vi "Plane Coordinate Generator.vi"(8 "error in (no error)":errorcluster, 10 "AcquireZplane Index":i32, 11 "AOL_Globals":T1={"Imaging Protocol"=enum."AOL Z-Stack", "Number of POI"=0, "Number of Miniscans"=0, "Number of Trials"=0, "Number of Cycles "=0, "# Averaged Frames"=0, "Laser power (%)"=0, "Pockels (V)"=0.0, "Acquisition Length (sec)"=0.0, "Fill time (us)"=0.0, "POI Dwell time (us)"=0.0, "Miniscan Dwell time per pixel (us)"=0.0, "PMT 1"=0.0, "PMT 2"=0.0, "Back Apperture (mA)"=512.0, "Frame Size"=0, "Center Frequency"=0.0, "Field of View (um)"=175.0, "Field of View (norm)"=0.0, "DwellTime (us)"=0.0, "Ref Dwell Time (us)"=0.0, "Wavelength (nm)"=0.0, "Zoom"=0.0, "AOL Z"=0.0, "AOL Mode"=enum."Raster", "GridXY"=0.0, "GridZ"=0.0, "TriggerPeriod (sec)"=0.0, "Number of Pixels in Miniscan"=0, "Experiment folder path"=path "", "X centre"=0.0, "Y centre"=0.0, "Angle (degrees)"=0.0, "Angle Xs (degrees)"=0.0, "Angle Ys (degrees)"=0.0, "Plane Mode"=0, "Threshold"=[], "Regenerate Chirps"=FALSE, "Rectangle ROI length (pixels)"=0, "Rectangle ROI height (pixels)"=0, "AOD fill"=4900, "StartupDelay"=0, "Samples Wait after Trigger"=5080, "Slip Cycle"=600000, "Add Cycle"=TRUE, "Functional Mode"=enum."Point", "Z Start"=0.0, "Z Stop"=0.0, "# Planes"=0, "Total Pixels"=0, "Variable Miniscan Pixels"=[], "Use Variable Length"=FALSE, "Use Variable Resolution"=FALSE, "Laser power (%) at Z Start"=0, "Laser power (%) at Z Stop"=0, "Ref Z Step"=0} {"Angle Ys (degrees)" format="%#.6g"; "Angle Xs (degrees)" format="%#.6g"; "Plane Mode" items=["XY Plane", "XZ Plane", "YZ Plane", "arbitraryplane"]; "Frame Size" items=["100X100"=100, "128X128"=128, "200X200"=200, "256X256"=256, "512X512"=512, "1024x1024"=1024, "2048x2048"=2048]; "Back Apperture (mA)" format="%#.6g"; "Pockels (V)" format="%#.6g"; "PMT 2" format="%#.6g"; "PMT 1" format="%#.6g"; "Angle (degrees)" format="%#.6g"; "POI Dwell time (us)" format="%#.6g"}) -> (0 "error out":errorcluster, 3 "ROI Attributes (broken down to miniscans)":T7)   [LabVIEW 2020]
uses:
  Typedefs/ROI XY coordinates cluster.ctl
  Typedefs/Controls/AOL_Globals.ctl
  Typedefs/Imaging Protocols enum.ctl
  Typedefs/Frame Size.ctl
  Typedefs/AOL modes.ctl
  Typedefs/Plane Mode.ctl
  Typedefs/Functional Mode.ctl
  User Interface/Visualisation/Functional Imaging Viewer/Typedefs/ROI parameters data type.ctl
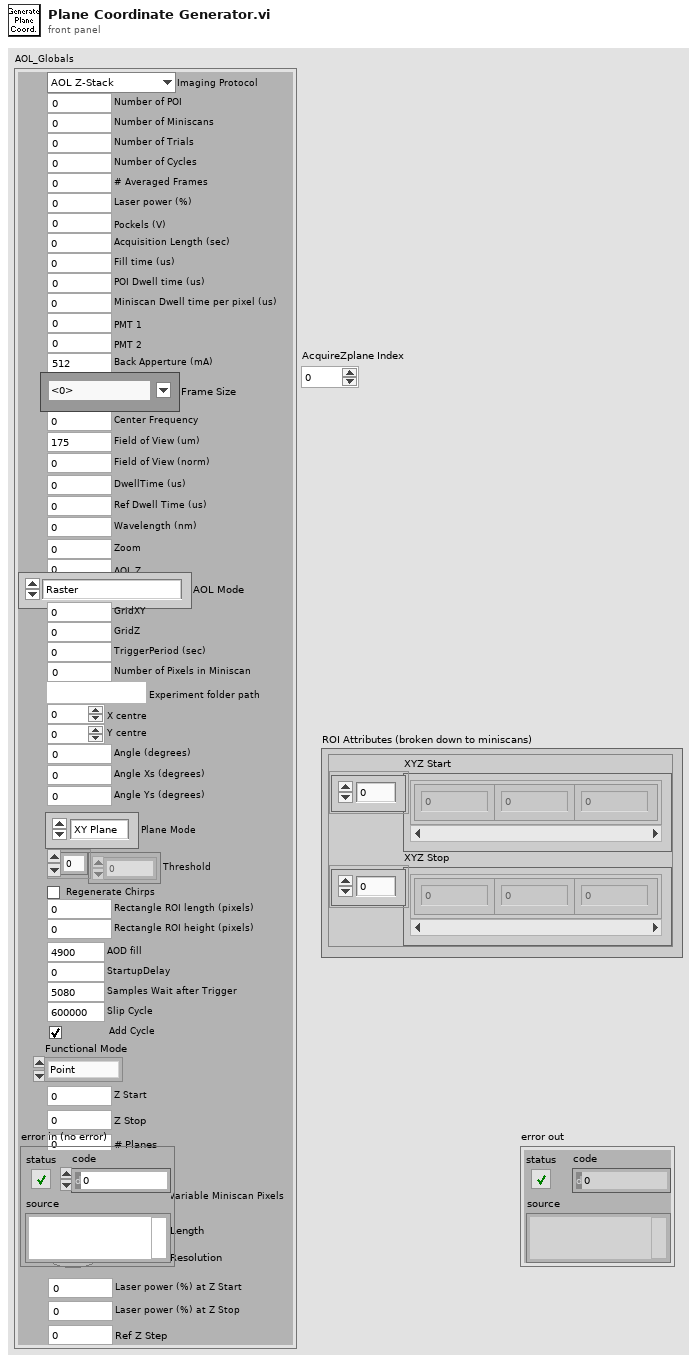
[diagram p1: front panel]
types:
  T1 = typedef "AOL_Globals.ctl" = cluster{"Imaging Protocol":T2, "Number of POI":u16, "Number of Miniscans":u16, "Number of Trials":u16, "Number of Cycles ":u64, "# Averaged Frames":u16, "Laser power (%)":u8, "Pockels (V)":dbl, "Acquisition Length (sec)":dbl, "Fill time (us)":dbl, "POI Dwell time (us)":dbl, "Miniscan Dwell time per pixel (us)":dbl, "PMT 1":dbl, "PMT 2":dbl, "Back Apperture (mA)":dbl, "Frame Size":T3, "Center Frequency":dbl, "Field of View (um)":dbl, "Field of View (norm)":dbl, "DwellTime (us)":dbl, "Ref Dwell Time (us)":dbl, "Wavelength (nm)":dbl, "Zoom":dbl, "AOL Z":dbl, "AOL Mode":T4, "GridXY":dbl, "GridZ":dbl, "TriggerPeriod (sec)":dbl, "Number of Pixels in Miniscan":u16, "Experiment folder path":path, "X centre":dbl, "Y centre":dbl, "Angle (degrees)":dbl, "Angle Xs (degrees)":dbl, "Angle Ys (degrees)":dbl, "Plane Mode":T5, "Threshold":u16[], "Regenerate Chirps":bool, "Rectangle ROI length (pixels)":u16, "Rectangle ROI height (pixels)":u16, "AOD fill":u16, "StartupDelay":i32, "Samples Wait after Trigger":u16, "Slip Cycle":u32, "Add Cycle":bool, "Functional Mode":T6, "Z Start":dbl, "Z Stop":dbl, "# Planes":i32, "Total Pixels":i32, "Variable Miniscan Pixels":u16[], "Use Variable Length":bool, "Use Variable Resolution":bool, "Laser power (%) at Z Start":u8, "Laser power (%) at Z Stop":u8, "Ref Z Step":i8}
  T2 = typedef "Imaging Protocols enum.ctl" = enum16{"AOL Z-Stack", "Motor Z Stack", "Parameter Sweep", "Functional Acquisition", "Single Plane Acquisition", "Volume Acquisition", "Live Imaging", "Live Plane Imaging", "Live Volume Imaging"}
  T3 = typedef "Frame Size.ctl" = u16
  T4 = typedef "AOL modes.ctl" = enum16{"Raster", "Structural", "Pointing", "Mini Scan", "Alignment"}
  T5 = typedef "Plane Mode.ctl" = u16
  T6 = typedef "Functional Mode.ctl" = enum16{"Point", "Line", "Patch", "Plane", "Volume"}
  T7 = typedef "ROI XY coordinates cluster.ctl" = cluster{"XYZ Start":cluster{"X":sgl, "Y":sgl, "Z":sgl}[], "XYZ Stop":cluster{"X":sgl, "Y":sgl, "Z":sgl}[]}
  T8 = typedef "ROI parameters data type.ctl" = cluster{"ROI index":dbl, "ROI ID":dbl, "ROI Time (ns)":dbl, "Pixels in ROI":dbl, "X start":dbl, "Y start":dbl, "Z start":dbl, "X stop":dbl, "Y stop":dbl, "Z stop":dbl, "Angle (deg)":dbl, "Composite ID":dbl, "Number of lines":dbl, "Frame Size":dbl, "Zoom":dbl, "Laser Power (%)":dbl, "ROI group ID":dbl, "Resolution":dbl, "Dwell Time per pixel":dbl, "Pixels per miniscan":dbl, "Original FOV (um)":dbl, "Apparent Frame Size":dbl, "Z Plane Idx":i32[], "Z Plane codes":i32[]}
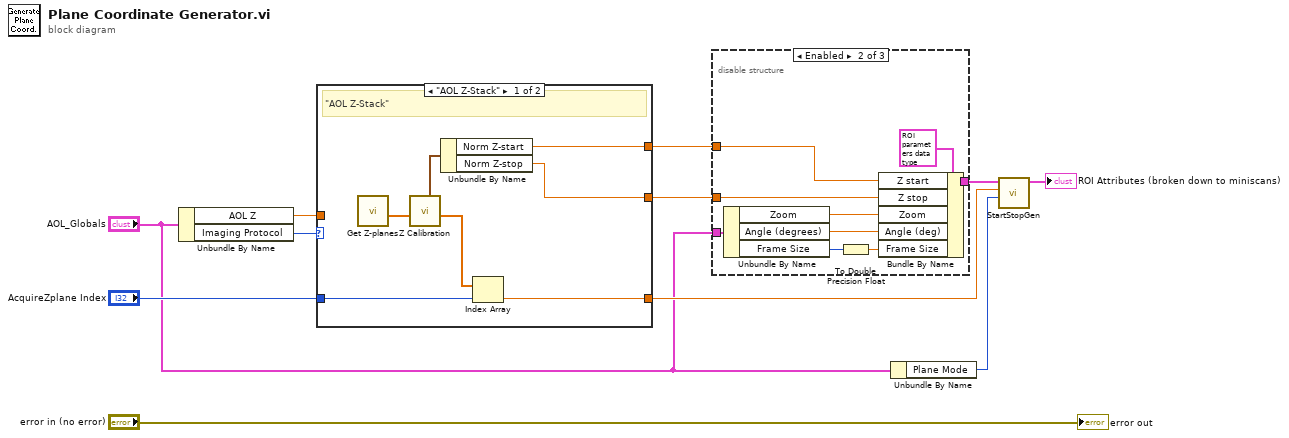
[diagram p0: block diagram]
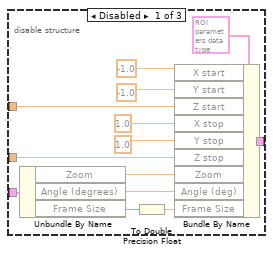
[diagram p2: hidden frame]
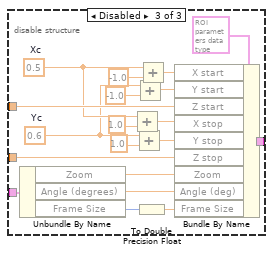
[diagram p3: hidden frame]
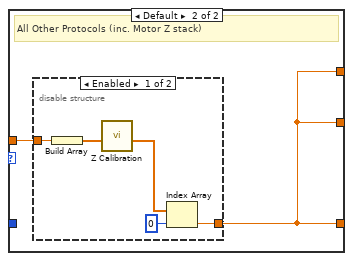
[diagram p4: hidden frame]
diagram:
  n1 = Unbundle By Name("AOL_Globals") -> ("AOL Z"=w3:dbl, "Imaging Protocol"=w4:T2)
  n2 = case shown="\"AOL Z-Stack\"" w4 {
    tunnel: [w12 w20] -> w10
    tunnel: [w13 w20] -> w9
    tunnel: "AcquireZplane Index" -> [w18 _]
    tunnel: [w17 w20] -> w6
    tunnel: w3 -> [_ w19]
    frame "AOL Z-Stack" {
      # "\"AOL Z-Stack\""
      n3 = call "Get Z-planes.vi"() -> ("Z Planes(um)"=w16:dbl[])  [unwired: 7 in, 4 out]
      n4 = call "Z Calibration.vi"("Z Planes"=w16) -> ("Norm Z"=w15:dbl[], "Norm Z start/stop"=w14:cluster{"Norm Z-start":dbl, "Norm Z-stop":dbl})  [unwired: 7 in, 2 out]
      n5 = Unbundle By Name(w14) -> ("Norm Z-start"=w13:dbl, "Norm Z-stop"=w12:dbl)
      n6 = Index Array(array=w15, index=w18) -> (element=w17:dbl)
    }
    frame Default {
      # "All Other Protocols (inc. Motor Z stack)"
      n7 = disable-structure shown="Enabled" {
        disable-tunnel: [w22 w26] -> w20
        disable-tunnel: w19 -> [w21 w26]
        frame Enabled {
          n8 = Build Array(w21) -> (w25:dbl[])
          n9 = call "Z Calibration.vi"("Z Planes"=w25) -> ("Norm Z"=w24:dbl[])  [unwired: 7 in, 3 out]
          n10 = Index Array(array=w24, index=0) -> (element=w22:dbl)
        }
        frame Disabled {
        }
      }
    }
  }
  n11 = disable-structure shown="Enabled" {
    disable-tunnel: w10 -> [w37 w48 w66]
    disable-tunnel: w9 -> [w36 w47 w65]
    disable-tunnel: [w35 w46 w64] -> w8
    disable-tunnel: "AOL_Globals" -> [w29 w40 w58]
    frame Disabled {
      n12 = Unbundle By Name(w29) -> ("Zoom"=w32:dbl, "Angle (degrees)"=w31:dbl, "Frame Size"=w30:T3)
      n13 = To Double Precision Float(number=w30) -> (double precision float=w33:dbl)
      n14 = Bundle By Name(cluster=T8 {"ROI index"=0.0, "ROI ID"=0.0, "ROI Time (ns)"=0.0, "Pixels in ROI"=0.0, "X start"=0.0, "Y start"=0.0, "Z start"=0.0, "X stop"=0.0, "Y stop"=0.0, "Z stop"=0.0, "Angle (deg)"=0.0, "Composite ID"=0.0, "Number of lines"=0.0, "Frame Size"=0.0, "Zoom"=0.0, "Laser Power (%)"=0.0, "ROI group ID"=0.0, "Resolution"=0.0, "Dwell Time per pixel"=0.0, "Pixels per miniscan"=0.0, "Original FOV (um)"=0.0, "Apparent Frame Size"=0.0, "Z Plane Idx"=[], "Z Plane codes"=[]} ("X-Y-Z coordinates"), "X start"=-1.0, "Y start"=-1.0 ("X start"), "Z start"=w36, "X stop"=1.0, "Y stop"=1.0 ("X stop"), "Z stop"=w37, "Zoom"=w32, "Angle (deg)"=w31, "Frame Size"=w33) -> (w35:T8)
    }
    frame Enabled {
      n15 = Unbundle By Name(w40) -> ("Zoom"=w43:dbl, "Angle (degrees)"=w42:dbl, "Frame Size"=w41:T3)
      n16 = To Double Precision Float(number=w41) -> (double precision float=w44:dbl)
      n17 = Bundle By Name(cluster=T8 {"ROI index"=0.0, "ROI ID"=0.0, "ROI Time (ns)"=0.0, "Pixels in ROI"=0.0, "X start"=0.0, "Y start"=0.0, "Z start"=0.0, "X stop"=0.0, "Y stop"=0.0, "Z stop"=0.0, "Angle (deg)"=0.0, "Composite ID"=0.0, "Number of lines"=0.0, "Frame Size"=0.0, "Zoom"=0.0, "Laser Power (%)"=0.0, "ROI group ID"=0.0, "Resolution"=0.0, "Dwell Time per pixel"=0.0, "Pixels per miniscan"=0.0, "Original FOV (um)"=0.0, "Apparent Frame Size"=0.0, "Z Plane Idx"=[], "Z Plane codes"=[]} ("X-Y-Z coordinates"), "Z start"=w47, "Z stop"=w48, "Zoom"=w43, "Angle (deg)"=w42, "Frame Size"=w44) -> (w46:T8)
    }
    frame Disabled {
      w49 = 0.6  # Yc
      w54 = 0.5  # Xc
      n18 = Unbundle By Name(w58) -> ("Zoom"=w61:dbl, "Angle (degrees)"=w60:dbl, "Frame Size"=w59:T3)
      n19 = Add(x=w54, y=1.0 ("X stop")) -> (x+y=w56:dbl)
      n20 = Add(x=w49, y=1.0 ("X stop")) -> (x+y=w52:dbl)
      n21 = Add(x=w49, y=-1.0 ("X start")) -> (x+y=w50:dbl)
      n22 = To Double Precision Float(number=w59) -> (double precision float=w62:dbl)
      n23 = Add(x=w54, y=-1.0 ("X start")) -> (x+y=w57:dbl)
      n24 = Bundle By Name(cluster=T8 {"ROI index"=0.0, "ROI ID"=0.0, "ROI Time (ns)"=0.0, "Pixels in ROI"=0.0, "X start"=0.0, "Y start"=0.0, "Z start"=0.0, "X stop"=0.0, "Y stop"=0.0, "Z stop"=0.0, "Angle (deg)"=0.0, "Composite ID"=0.0, "Number of lines"=0.0, "Frame Size"=0.0, "Zoom"=0.0, "Laser Power (%)"=0.0, "ROI group ID"=0.0, "Resolution"=0.0, "Dwell Time per pixel"=0.0, "Pixels per miniscan"=0.0, "Original FOV (um)"=0.0, "Apparent Frame Size"=0.0, "Z Plane Idx"=[], "Z Plane codes"=[]} ("X-Y-Z coordinates"), "X start"=w57, "Y start"=w50, "Z start"=w65, "X stop"=w56, "Y stop"=w52, "Z stop"=w66, "Zoom"=w61, "Angle (deg)"=w60, "Frame Size"=w62) -> (w64:T8)
    }
  }
  n25 = Unbundle By Name("AOL_Globals") -> ("Plane Mode"=w2:T5)
  n26 = call "StartStopGen.vi"("PlaneMode"=w2, "AOLZ"=w6, "X-Y-Z coordinates"=w8) -> ("ROI Coordinates (broken down to miniscans)"=→"ROI Attributes (broken down to miniscans)":T7)  [unwired: 8 in]
  "error out" <- "error in (no error)"
